vi "ObtainMainQueue.vi"(8 "ErrorIn":errorcluster caption="エラー入力（エラーなし）", 11 "QName":string) -> (0 "ErrorOut":errorcluster caption="エラー出力", 2 "SampleQ":cluster{"Status":T1, "Data":variant}, 3 "QueueOut":refnum<queue>)   [LabVIEW 2021]
doc: "SP1TaskLoop および、SP2TaskLoop へコマンドを送信するキューを作成します。\nキューに入れるデータは、コマンド（StepName）とデータ（Data）の入ったクラスタです。"
uses:
  MainStatus.ctl
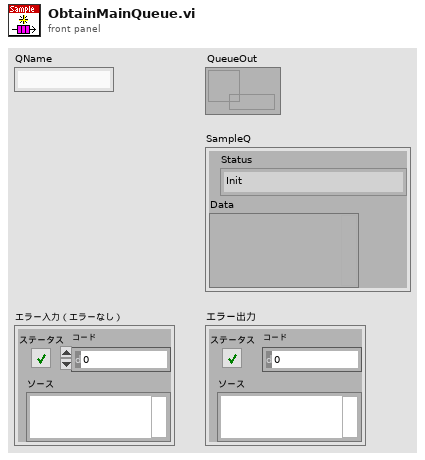
[diagram p1: front panel]
types:
  T1 = typedef "MainStatus.ctl" = enum16{"Init", "Status", "Placed", "Setting", "Start", "Data", "Collected", "Quit"}
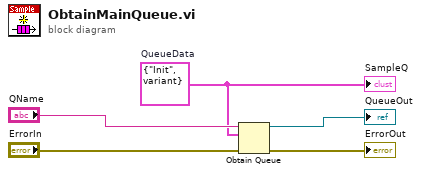
[diagram p0: block diagram]
diagram:
  w3 = cluster{"Status":T1, "Data":variant} {"Status"=enum."Init", "Data"=variant}  # QueueData
  n1 = Obtain Queue(name (unnamed)="QName", element data type=w3, error in (no error)="ErrorIn") -> (queue out=→"QueueOut":refnum<queue>, error out=→"ErrorOut":errorcluster)  [unwired: 2 in, 1 out]
  "SampleQ" <- w3
